vi "MenuActivation Response.vi"(8 "error in (no error)":errorcluster, 9 "Coords":T1, 10 "Menu Refnum":refnum<k9>, 11 "UEF Handler1 in":refnum<class "UEF Handler2.lvclass">) -> (0 "error out":errorcluster, 3 "UEF Handler1 out":refnum<class "UEF Handler2.lvclass">)   [LabVIEW 2015, in "UEF Handler2.lvclass"]
uses:
  UEF Handler2.lvclass
  <vilib>/Utility/miscctls.llb/LVPoint32TypeDef.ctl
  <vilib>/LIEF/Image Editor Handler/Image Editor Handler.lvclass/Image Editor Handler.ctl
  <vilib>/LIEF/Image Editor Handler/Read PictureRef.vi
  <vilib>/LIEF/Image Editor Handler/Read Shapes.vi
  <vilib>/LIEF/Forms/Shape/Shape.lvclass
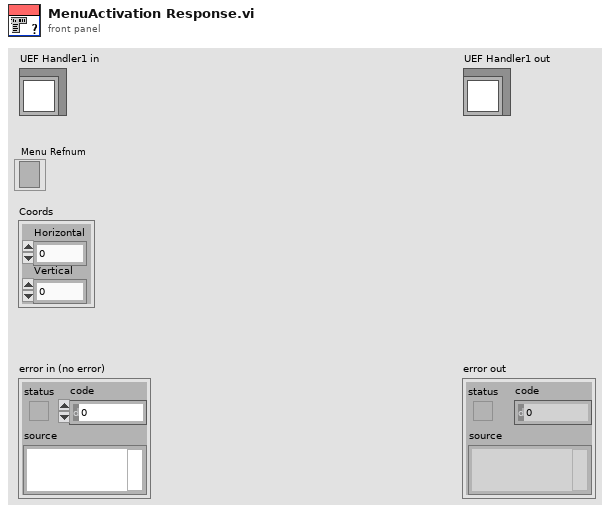
[diagram p1: front panel]
types:
  T1 = typedef "LVPoint32TypeDef.ctl" = cluster{"Horizontal":i32, "Vertical":i32}
  T2 = typedef "LVPositionTypeDef.ctl" = cluster{"Left":i32, "Top":i32}
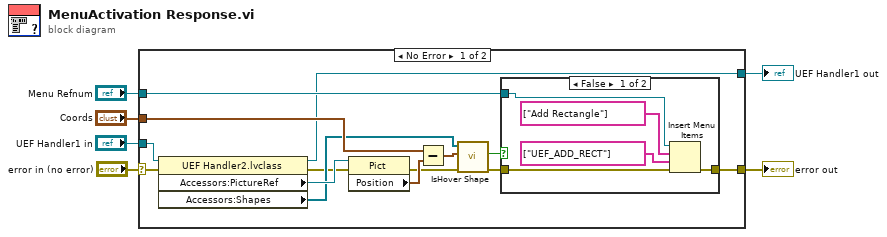
[diagram p0: block diagram]
diagram:
  n1 = case shown="No Error" "error in (no error)" {
    selector: "error in (no error)" -> [w7 w27]
    tunnel: "UEF Handler1 in" -> [w20 w28]
    tunnel: "Coords" -> [w18 _]
    tunnel: "Menu Refnum" -> [w13 _]
    tunnel: [w12 w28] -> w2
    tunnel: [w11 w27] -> w1
    frame No Error {
      n2 = property class="UEF Handler2.lvclass"(reference=w20, error in=w7) -> (reference out=w12:refnum<class "UEF Handler2.lvclass">, error out=w8:errorcluster, "Accessors:PictureRef"=w19:refnum<vi>, "Accessors:Shapes"=w15:refnum<data-value>[])
      n3 = property class="Pict"(reference=w19, error in=w8) -> (error out=w9:errorcluster, "Position"=w17:T2)  [unwired: 1 out]
      n4 = Subtract(x=w18, y=w17) -> (x-y=w16:T1)
      n5 = call <vilib>:"IsHover Shape.vi"("error in (no error)"=w9, "Coords"=w16, "Shape in"=w15) -> ("error out"=w10:errorcluster, "Found?"=w14:bool)  [unwired: 3 in, 4 out]
      n6 = case shown="False" w14 {
        tunnel: w13 -> [w25 _]
        tunnel: [w22 w26] -> w11
        tunnel: w10 -> [w21 w26]
        frame False {
          n7 = Insert Menu Items(6:w21, 7:string[] ["UEF_ADD_RECT"] ("item names"), 8:string[] ["Add Rectangle"] ("item names"), 9:w25) -> (0:w22:errorcluster)  [unwired: 2 in, 2 out]
        }
        frame True {
        }
      }
    }
    frame Error {
    }
  }
  "error out" <- w1
  "UEF Handler1 out" <- w2
